vi "Actuator Controls 2 Array.vi"(10 "Actuator Controls":T1 {"Actuator Z2" min=-10.0 max=10.0 step=0.1 scale=-10.0..10.0; "Actuator Z3" min=-10.0 max=10.0 step=0.1 scale=-10.0..10.0; "Actuator X2" min=-10.0 max=10.0 step=0.1 scale=-10.0..10.0; "Actuator Y1" min=-10.0 max=10.0 step=0.1 scale=-10.0..10.0; "Actuator Z1" min=-10.0 max=10.0 step=0.1 scale=-10.0..10.0; "Actuator X1" min=-10.0 max=10.0 step=0.1 scale=-10.0..10.0}) -> (2 "Array":dbl[](array[numeric]))   [LabVIEW 2009]
uses:
  Actuator Controls.ctl
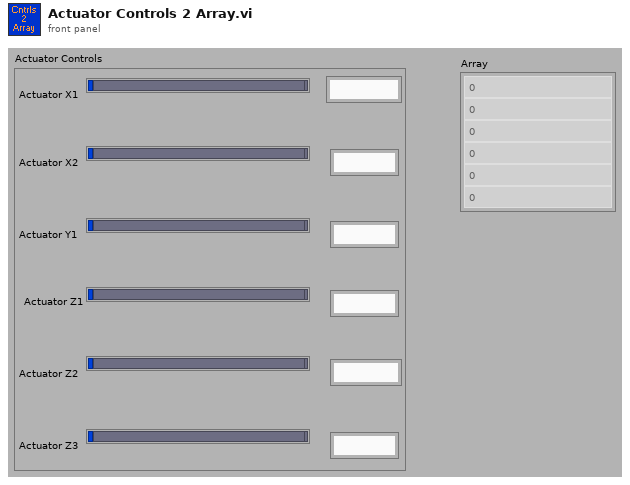
[diagram p1: front panel]
types:
  T1 = typedef "Actuator Controls.ctl" = cluster{"Actuator X1":dbl, "Actuator X2":dbl, "Actuator Y1":dbl, "Actuator Z1":dbl, "Actuator Z2":dbl, "Actuator Z3":dbl}
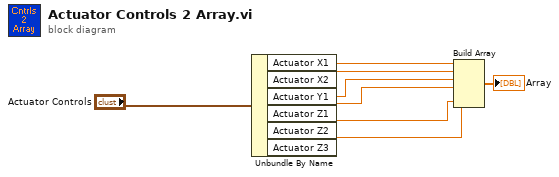
[diagram p0: block diagram]
diagram:
  n1 = Unbundle By Name("Actuator Controls") -> ("Actuator X1"=w3:dbl, "Actuator X2"=w4:dbl, "Actuator Y1"=w5:dbl, "Actuator Z1"=w6:dbl, "Actuator Z2"=w7:dbl, "Actuator Z3"=w8:dbl)
  n2 = Build Array(w3, w4, w5, w6, w7, w8) -> (→"Array":dbl[])
